vi "Purge.vi"(8 "Purge":bool, 10 "Fuel Arm":bool, 11 "Engine Arm":bool) -> (0 "Solenoids":bool[](array[boolean]))   [LabVIEW 2016]
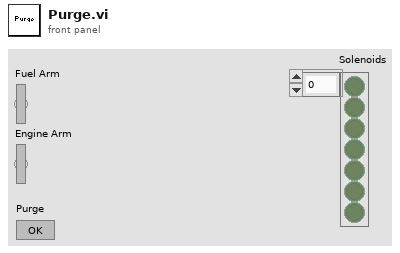
[diagram p1: front panel]
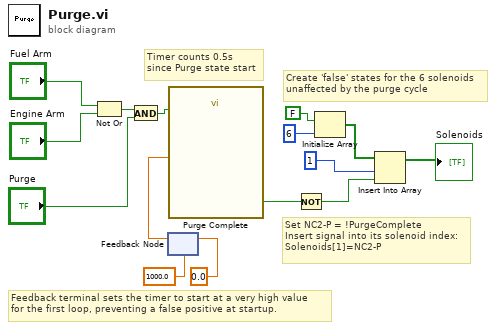
[diagram p0: block diagram]
diagram:
  # "Feedback terminal sets the timer to start at a very high value \nfor the first loop, preventing a false positive at startup."
  # "Timer counts 0.5s\nsince Purge state start"
  # "Set NC2-P = !PurgeComplete\nInsert signal into its solenoid index:\nSolenoids[1]=NC2-P"
  # "Create 'false' states for the 6 solenoids\nunaffected by the purge cycle"
  n1 = Not Or(1:"Engine Arm", 2:"Fuel Arm") -> (0:w13:bool)
  n2 = And(x=w13, y="Purge") -> (x .and. y?=w12:bool)
  n3 = feedback #1(1000.0) -> (w2:dbl)
  n4 = feedback-in #1(0.0) -> ()
  n5 = call "Purge Complete"("Reset"=w12, "Set Start Time (s)"=w2) -> ("Time has Elapsed"=w11:bool)  [unwired: 10 in, 7 out]
  n6 = Not(x=w11) -> (.not. x?=w7:bool)
  n7 = Initialize Array(FALSE, 6) -> (w8:bool[])
  n8 = Insert Into Array(array=w8, index=1, new element=w7) -> (→"Solenoids":bool[])
